vi "Update.vi"(8 "error in (no error)":errorcluster, 11 "Dual Fan in":refnum<class "Dual Fan.lvclass">) -> (0 "error out":errorcluster, 3 "Dual Fan out":refnum<class "Dual Fan.lvclass">)   [LabVIEW 2012, in "Dual Fan.lvlib" / "Dual Fan.lvclass"]
uses:
  Dual Fan.lvclass
  Simulation/Simulation Data_Global.vi
  Simulation/Simulation.lvlib
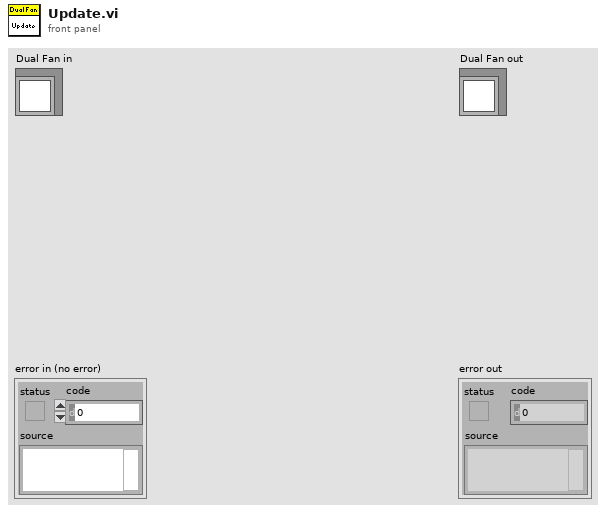
[diagram p1: front panel]
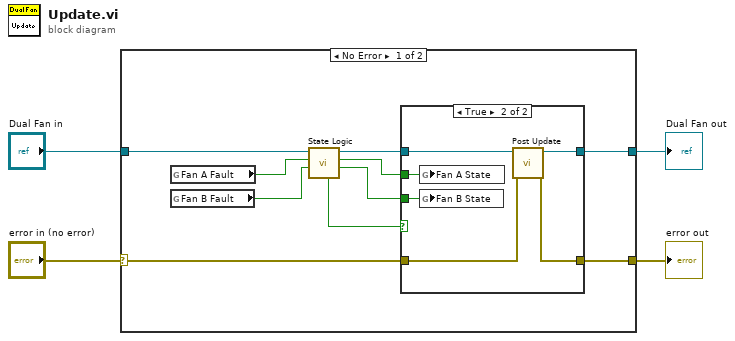
[diagram p0: block diagram]
diagram:
  n1 = case shown="No Error" "error in (no error)" {
    selector: "error in (no error)" -> [w14 w24]
    tunnel: [w12 w24] -> w3
    tunnel: [w13 w23] -> w1
    tunnel: "Dual Fan in" -> [w11 w23]
    frame No Error {
      n2 = global read "Simulation Data_Global.vi" "Fan A Fault"() -> (w5:bool)
      n3 = global read "Simulation Data_Global.vi" "Fan B Fault"() -> (w6:bool)
      n4 = call "State Logic.vi"("Fan B Fault"=w6, "Fan A Fault"=w5, "Dual Fan in"=w11) -> ("Fan B State"=w8:bool, "Fan A State"=w9:bool, "Dual Fan out"=w10:refnum<class "Dual Fan.lvclass">, "Changed?"=w7:bool)  [unwired: 5 in]
      n5 = case shown="True" w7 {
        tunnel: w14 -> [w15 w22]
        tunnel: [w16 w21] -> w13
        tunnel: [w15 w20] -> w12
        tunnel: w10 -> [w16 w19]
        tunnel: w9 -> [_ w18]
        tunnel: w8 -> [_ w17]
        frame False {
        }
        frame True {
          n6 = global write "Simulation Data_Global.vi" "Fan A State"(w18) -> ()
          n7 = global write "Simulation Data_Global.vi" "Fan B State"(w17) -> ()
          n8 = call "Post Update.vi"("error in (no error)"=w22, "Dual Fan in"=w19) -> ("error out"=w20:errorcluster, "Dual Fan out"=w21:refnum<class "Dual Fan.lvclass">)  [unwired: 8 in]
        }
      }
    }
    frame Error {
    }
  }
  "error out" <- w3
  "Dual Fan out" <- w1
